vi "DIMPowerSupply.ProcEvents.vi"(0 "i ref in":refnum<vi>, 5 "error in (no error)":errorcluster) -> (14 "i ref out":refnum<vi>, 19 "error out":errorcluster)   [LabVIEW 2014, in "DIMPowerSupply.lvlib"]
doc: "This method is used to define the events the object will listen to. Add your own events here."
uses:
  DIMPowerSupply.lvlib
  CSCore/CAEObj/CAEObj.event definition.ctl
  CSCore/BaseProcess/BaseProcess.event definition.ctl
  CSCore/BaseProcess/BaseProcess.descriptor string definition.ctl
  CSCore/BaseProcess/BaseProcess.lvlib
  CSCore/CAEObj/CAEObj.lvlib
panel:
  in  "event definition type":T1
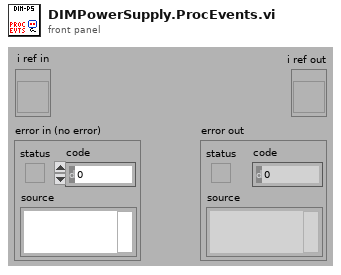
[diagram p1: front panel]
types:
  T1 = typedef "CAEObj.lvlib/CAEObj.event definition.ctl" = cluster{"URL":string, "enable":bool, "ignoreResID":bool}
  T2 = typedef "BaseProcess.lvlib/BaseProcess.event definition.ctl" = cluster{"CAEEvtDef":T1, "Data Descriptor":T3}
  T3 = typedef "BaseProcess.lvlib/BaseProcess.descriptor string definition.ctl" = string
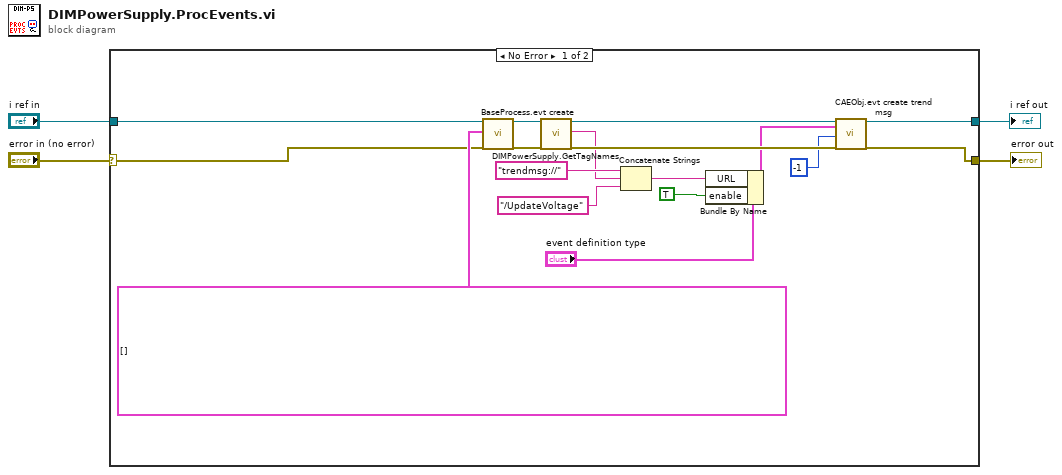
[diagram p0: block diagram]
diagram:
  n1 = case shown="No Error" "error in (no error)" {
    selector: "error in (no error)" -> [w5 w22]
    tunnel: "i ref in" -> [w21 w23]
    tunnel: [w17 w23] -> w3
    tunnel: [w16 w22] -> w2
    frame No Error {
      n2 = call "BaseProcess.evt create.vi"("i ref in"=w21, "newEvents"=T2[] [] ("new events"), "error in (no error)"=w5) -> ("i ref out"=w13:refnum<vi>, "error out"=w12:errorcluster)  [unwired: 13 in, 2 out]
      n3 = call "DIMPowerSupply.GetTagNames.vi"("i ref in"=w13, "error in (no error)"=w12) -> ("i ref out"=w20:refnum<vi>, "MonTagName"=w6:string, "error out"=w19:errorcluster)  [unwired: 14 in, 1 out]
      n4 = Concatenate Strings("trendmsg://" ("string"), w6, "/UpdateVoltage" ("string")) -> (w10:string)
      n5 = Bundle By Name(cluster="event definition type", "URL"=w10, "enable"=TRUE) -> (w8:T1)
      n6 = call "CAEObj.evt create trend msg.vi"("i ref in"=w20, "event definition"=w8, "ms timeout (10000)"=-1 ("ms timeout (100)"), "error in (no error)"=w19) -> ("i ref out"=w17:refnum<vi>, "error out"=w16:errorcluster)  [unwired: 12 in, 2 out]
    }
    frame Error {
    }
  }
  "i ref out" <- w3
  "error out" <- w2
